vi "Preprocess Command.vi"(8 "error in (no error)":errorcluster, 10 "Command":string) -> (0 "error out":errorcluster, 2 "Arguments":string[](array[string]), 3 "Command":T1)   [LabVIEW 2017]
uses:
  Type Definitions/Command.ctl
  <vilib>/Utility/error.llb/Error Cluster From Error Code.vi
  <vilib>/ErrorRing/Error Ring.xnode
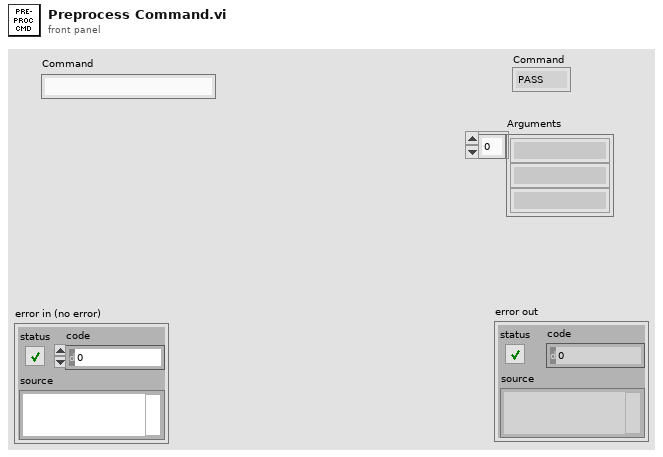
[diagram p1: front panel]
types:
  T1 = typedef "Command.ctl" = enum16{"PASS", "COPY"}
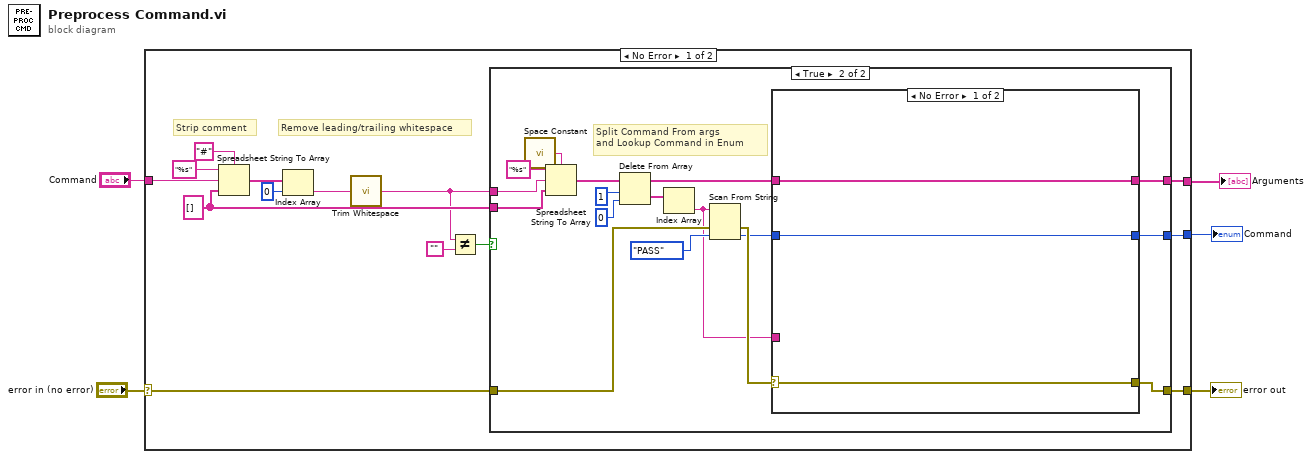
[diagram p0: block diagram]
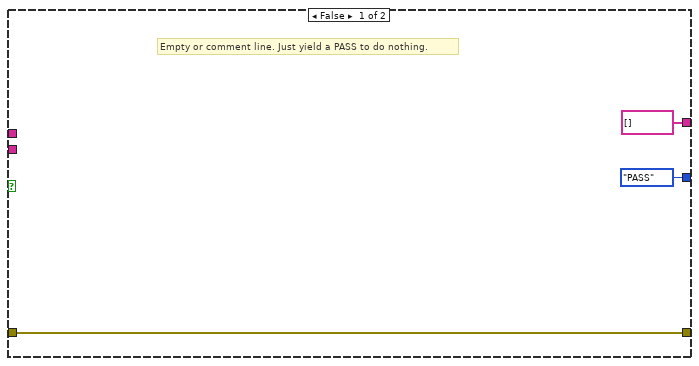
[diagram p2: hidden frame]
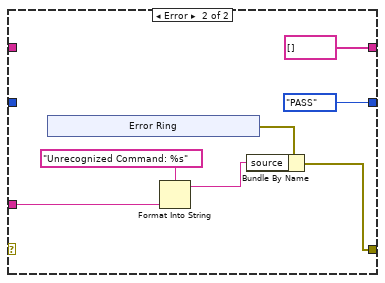
[diagram p3: hidden frame]
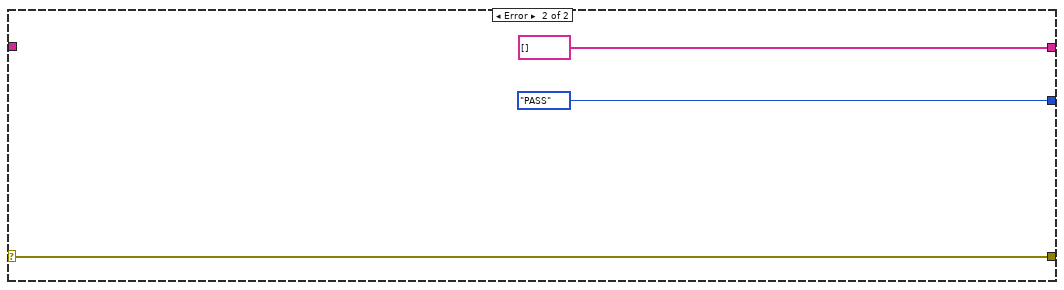
[diagram p4: hidden frame]
diagram:
  n1 = case shown="No Error" "error in (no error)" {
    selector: "error in (no error)" -> [w12 w54]
    tunnel: "Command" -> [w16 _]
    tunnel: [w9 string[] []] -> w4
    tunnel: [w10 w54] -> w3
    tunnel: [w11 Command."PASS" ("Command 2")] -> w2
    frame No Error {
      w14 = string[] []
      # "Remove leading/trailing whitespace"
      # "Strip comment"
      n2 = Spreadsheet String To Array(delimiter (Tab)="#", format string="%s", spreadsheet string=w16, array type (2D Dbl)=w14) -> (array=w18:string[])
      n3 = Index Array(array=w18, index=0) -> (element=w15:string)
      n4 = call <vilib>:"Trim Whitespace.vi"("string"=w15) -> ("trimmed string"=w6:string)  [unwired: 1 in]
      n5 = Not Equal?(x=w6, y="") -> (x != y?=w8:bool)
      n6 = case shown="True" w8 {
        tunnel: w6 -> [_ w39]
        tunnel: w14 -> [_ w37]
        tunnel: w12 -> [w20 w30]
        tunnel: [Command."PASS" ("Command 2") w27] -> w11
        tunnel: [w20 w26] -> w10
        tunnel: [string[] [] w24] -> w9
        frame False {
          # "Empty or comment line. Just yield a PASS to do nothing."
        }
        frame True {
          # "Split Command From args\nand Lookup Command in Enum"
          n7 = call <vilib>:"Space Constant.vi"() -> ("String"=w38:string)
          n8 = Spreadsheet String To Array(delimiter (Tab)=w38, format string="%s", spreadsheet string=w39, array type (2D Dbl)=w37) -> (array=w36:string[])
          n9 = Delete From Array(array=w36, length=1, index=0) -> (deleted portion=w33:string[], array with subset deleted=w25:string[])
          n10 = Index Array(array=w33) -> (element=w23:string)  [unwired: 1 in]
          n11 = Scan From String(input string=w23, error in=w30, default 1=Command."PASS" ("Command 2")) -> (error out=w29:errorcluster, output 1=w28:T1)  [unwired: 2 in, 2 out]
          n12 = case shown="No Error" w29 {
            selector: w29 -> [w41 _]
            tunnel: w28 -> [w42 _]
            tunnel: [w42 Command."PASS" ("Command 2")] -> w27
            tunnel: [w41 w46] -> w26
            tunnel: w25 -> [w40 _]
            tunnel: [w40 string[] []] -> w24
            tunnel: w23 -> [_ w44]
            frame No Error {
            }
            frame Error {
              n13 = xnode "Error Ring"() -> ("error out"=w47:errorcluster)
              n14 = Format Into String(format string="Unrecognized Command: %s", w44) -> (resulting string=w43:string)  [unwired: 2 in, 1 out]
              n15 = Bundle By Name(cluster=w47, "source"=w43) -> (w46:errorcluster)
            }
          }
        }
      }
    }
    frame Error {
    }
  }
  "Arguments" <- w4
  "Command" <- w2
  "error out" <- w3
